vi "Stop.vi"(6 "Teller":T1 {"AbsoluteTime" format="%<%x %.3X>T"}, 8 "Error in":errorcluster, 11 "Base Actor in":refnum<class "BaseActor.lvclass">) -> (0 "Error out":errorcluster, 3 "Base Actor out":refnum<class "BaseActor.lvclass">)   [LabVIEW 2020, in "jettl.lvlib" / "BaseActor.lvlib" / "BaseActor.lvclass"]
uses:
  BaseActor.lvclass
  BaseActor.lvclass/BaseActor.ctl
  jettl.lvlib
  Lifetime.ctl
  MessageMetadata.ctl
  TellOrigin.ctl
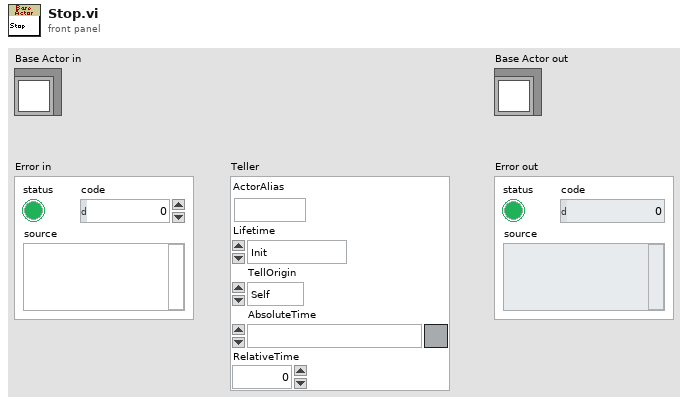
[diagram p1: front panel]
types:
  T1 = typedef "jettl.lvlib/MessageMetadata.ctl" = cluster{"ActorAlias":string, "Lifetime":T2, "TellOrigin":T3, "AbsoluteTime":timestamp, "RelativeTime":dbl}
  T2 = typedef "jettl.lvlib/Lifetime.ctl" = enum16{"Init", "Spawn", "Setup", "TeardownBeforeRunning", "Running", "StopCalled", "StoppingWithComponents", "StoppingNoComponents", "TeardownAfterRunning", "Stopped"}
  T3 = typedef "jettl.lvlib/TellOrigin.ctl" = enum16{"Self", "Mediator", "Component"}
  T4 = typedef "jettl.lvlib/Lifetime.ctl" = enum16{"Init", "Spawn", "Setup", "Teardown Before Running", "Running", "Stop Called", "Stopping With Children", "Stopping Without Children", "Teardown After Running", "Stopped"}
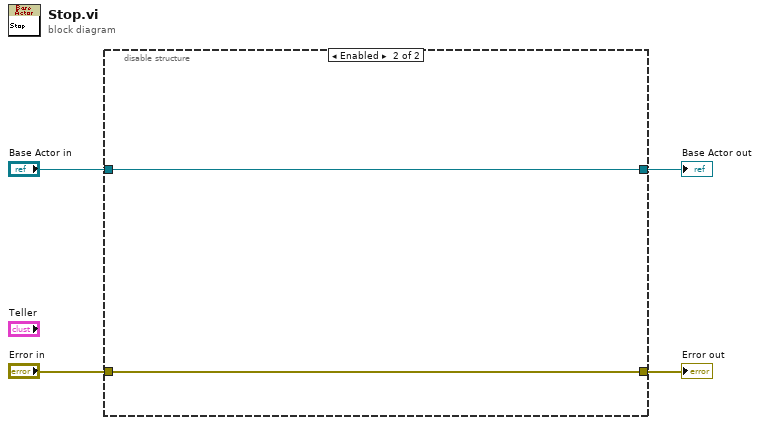
[diagram p0: block diagram]
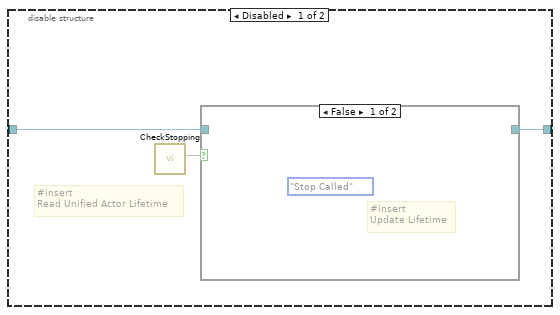
[diagram p2: hidden frame]
diagram:
  n1 = disable-structure shown="Enabled" {
    disable-tunnel: [w8 w14] -> w4
    disable-tunnel: "Base Actor in" -> [w6 w14]
    disable-tunnel: [_ w13] -> w2
    disable-tunnel: "Error in" -> [_ w13]
    frame Disabled {
      # "#insert\nRead Unified Actor Lifetime"
      n2 = call "CheckStopping.vi"() -> (2:w7, 10:w5)  [unwired: 9 in, 1 out]
      n3 = case shown="False" w7 {
        tunnel: w6 -> [w10 w12]
        tunnel: [w9 w12] -> w8
        frame False {
          w11 = Lifetime."Stop Called" ("Lifetime")
          # "#insert\nUpdate Lifetime"
        }
        frame True {
        }
      }
    }
    frame Enabled {
    }
  }
  "Base Actor out" <- w4
  "Error out" <- w2
